vi "LVClass_HasoEngine Get Preferences.vi"(0 "HasoEngine in":refnum<class "HasoEngine.lvclass">, 11 "error in (no error)":errorcluster) -> (4 "HasoEngine out":refnum<class "HasoEngine.lvclass">, 6 "Slopes engine setup":T1={"Start sub-aperture"={"X"=0, "Y"=0}, "Pupil average"=670.0} {"Pupil average" min=0.0 max=1.0}, 15 "error out":errorcluster)   [LabVIEW 2020, in "HasoEngine.lvclass"]
doc: "HasoSlopes computation preferences getter.\n\n--------------------------------------------------------------------------------\n\n<B>HasoEngineIn </B> : HasoEngine object.\n<B>HasoEngineOut </B> : HasoEngine object.\n<B>start_subpupil </B> : Coordinates of the first calculated sub-pupil (index coordinates relative to\n the top-left corner of the pupil).\n<B>denoising_strength </B> : Sensitivity of spot detection on summed images (between 0 and 1).\n<B>ErrorIn </B> : Error\n<B>ErrorOut </B> : Error\n\n--------------------------------------------------------------------------------"
uses:
  HasoEngine.lvclass
  SlopesEngineSetup.ctl
  Point2D.ctl
  HasoEngine.lvclass/HasoEngine.ctl
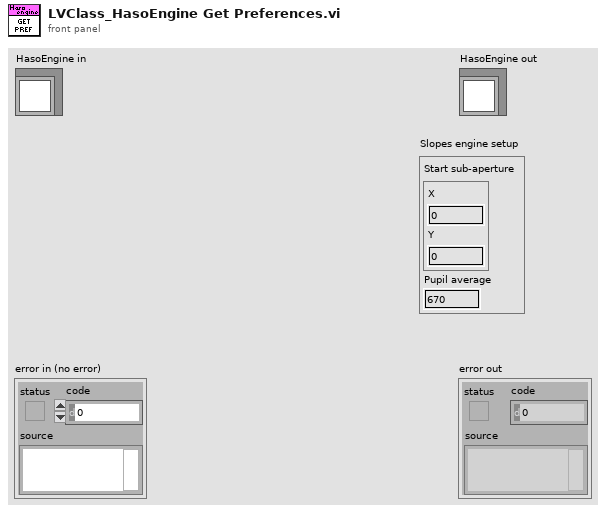
[diagram p1: front panel]
types:
  T1 = typedef "SlopesEngineSetup.ctl" = cluster{"Start sub-aperture":T2, "Pupil average":dbl}
  T2 = typedef "Point2D.ctl" = cluster{"X":u32, "Y":u32}
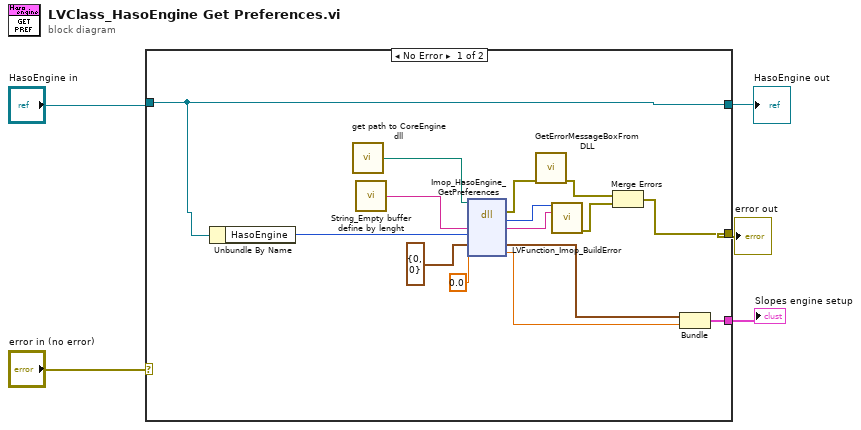
[diagram p0: block diagram]
diagram:
  n1 = case shown="No Error" "error in (no error)" {
    selector: "error in (no error)" -> [_ w21]
    tunnel: "HasoEngine in" -> [w10 w22]
    tunnel: [w10 w22] -> w2
    tunnel: [w6 w21] -> w3
    tunnel: [w11 _] -> w1
    frame No Error {
      n2 = Unbundle By Name(w10) -> ("HasoEngine"=w9:i32)
      n3 = call "get path to CoreEngine dll.vi"() -> ("path to c_interface_vc100.dll"=w17:path)  [unwired: 12 in, 3 out]
      n4 = call "String_Empty buffer define by lenght.vi"() -> ("Empty buffer"=w18:string)  [unwired: 1 in]
      n5 = dll-call lib="D:/2_trunk/Soft_haso/ImOpCoreEngine4_LV2011/DLLs/ImopEngine4_vc100.dll" fn="Imop_HasoEngine_GetPreferences"(path in=w17, "message"=w18, "objet"=w9, "StartSubPupil"=T2 {"X"=0, "Y"=0} ("dimension 2"), "pupil_average"=sgl 0.0) -> (error out=w16:errorcluster, "return type"=w19:i32, "message"=w20:string, "StartSubPupil"=w13:T2, "pupil_average"=w12:sgl)  [unwired: 3 in, 1 out]
      n6 = call "GetErrorMessageBoxFromDLL.vi"("error IN"=w16) -> ("error OUT"=w8:errorcluster)  [unwired: 10 in]
      n7 = call "LVFunction_Imop_BuildError.vi"("code"=w19, "String to Prepend to source (\"\")"=w20) -> ("error out"=w7:errorcluster)  [unwired: 13 in]
      n8 = Merge Errors(w8, w7) -> (w6:errorcluster)
      n9 = Bundle("StartSubPupil"=w13, "pupil_average"=w12) -> (w11:cluster{"StartSubPupil":T2, "pupil_average":sgl})  [unwired: 1 in]
    }
    frame Error {
    }
  }
  "error out" <- w3
  "HasoEngine out" <- w2
  "Slopes engine setup" <- w1
